vi "Equipment.vi"() -> ()   [LabVIEW 2012]
uses:
  CalibrationTime.ctl
  Calibration_SN.ctl
  Calibration.ctl
panel:
  in  "Complete":bool
  in  "Calibration ID":T1
  in  "SN":T2
  in  "Calibration\nDue Date":T3 {"Eq20" format="%<%x>T"; "Eq19" format="%<%x>T"; "Eq18" format="%<%x>T"; "Eq17" format="%<%x>T"; "Eq16" format="%<%x>T"; "Eq15" format="%<%x>T"; "Eq14" format="%<%x>T"; "Eq13" format="%<%x>T"; "Eq12" format="%<%x>T"; "Eq11" format="%<%x>T"; "Eq10" format="%<%x>T"; "Eq9" format="%<%x>T"; "Eq8" format="%<%x>T"; "Eq7" format="%<%x>T"; "Eq6" format="%<%x>T"; "Eq5" format="%<%x>T"; "Eq4" format="%<%x>T"; "Eq3" format="%<%x>T"; "Eq2" format="%<%x>T"; "Eq1" format="%<%x>T"}
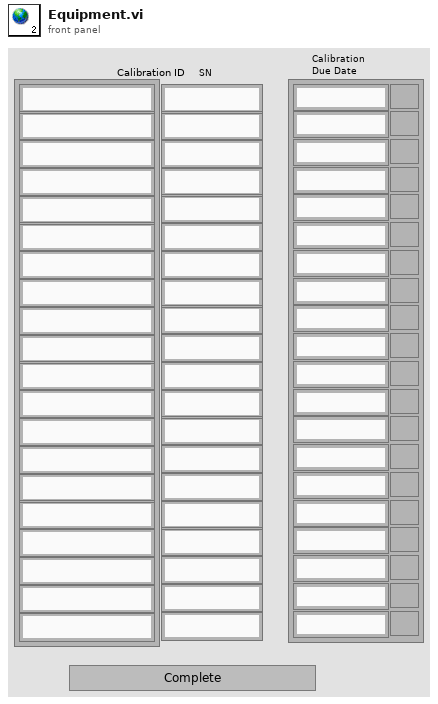
[diagram p1: front panel]
types:
  T1 = typedef "Calibration.ctl" = cluster{"Eq1":string, "Eq2":string, "Eq3":string, "Eq4":string, "Eq5":string, "Eq6":string, "Eq7":string, "Eq8":string, "Eq9":string, "Eq10":string, "Eq11":string, "Eq12":string, "Eq13":string, "Eq14":string, "Eq15":string, "Eq16":string, "Eq17":string, "Eq18":string, "Eq19":string, "Eq20":string}
  T2 = typedef "Calibration_SN.ctl" = cluster{"Eq1":string, "Eq2":string, "Eq3":string, "Eq4":string, "Eq5":string, "Eq6":string, "Eq7":string, "Eq8":string, "Eq9":string, "Eq10":string, "Eq11":string, "Eq12":string, "Eq13":string, "Eq14":string, "Eq15":string, "Eq16":string, "Eq17":string, "Eq18":string, "Eq19":string, "Eq20":string}
  T3 = typedef "CalibrationTime.ctl" = cluster{"Eq1":timestamp, "Eq2":timestamp, "Eq3":timestamp, "Eq4":timestamp, "Eq5":timestamp, "Eq6":timestamp, "Eq7":timestamp, "Eq8":timestamp, "Eq9":timestamp, "Eq10":timestamp, "Eq11":timestamp, "Eq12":timestamp, "Eq13":timestamp, "Eq14":timestamp, "Eq15":timestamp, "Eq16":timestamp, "Eq17":timestamp, "Eq18":timestamp, "Eq19":timestamp, "Eq20":timestamp}
diagram:
